vi "SR7265 _Set_V_OSC_ver1.0.vi"(0 "GPIB ADR":u16, 1 "Vosc Setpt":dbl format="%#_6e", 2 "error in":errorcluster) -> (3 "dump GPIB ADR":u16, 4 "dup Vosc Setpt":dbl format="%#_6e", 6 "error out":errorcluster)   [LabVIEW 2012]
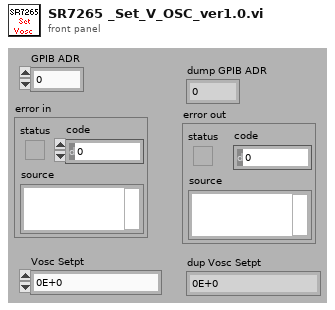
[diagram p1: front panel]
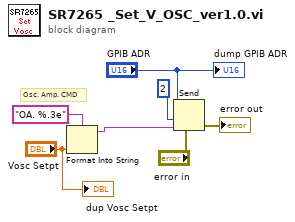
[diagram p0: block diagram]
diagram:
  # "Osc. Amp. CMD"
  n1 = Format Into String(format string="OA. %.3e", "Vosc Setpt") -> (resulting string=w3:string)  [unwired: 2 in, 1 out]
  n2 = Send(2:"GPIB ADR", 3:i16 2 ("mode"), 4:"error in", 5:w3) -> (8:→"error out":errorcluster)  [unwired: 1 in, 2 out]
  "dup Vosc Setpt" <- "Vosc Setpt"
  "dump GPIB ADR" <- "GPIB ADR"
